vi "Create Minor Grid Lines.vi"(0 "Major Count":u16, 1 "Axis":enum16{"X-Axis", "Y-Axis", "Z-Axis"}(ring), 2 "Grid Plane Visible":T1, 5 "Minor Count":u16, 7 "Range":cluster{"Max":sgl, "Min":sgl}, 9 "Grid Color":u32(colorbox), 11 "error in (no error)":errorcluster, 12 "Inverted?":bool, 13 "Logarithm?":bool) -> (4 "Grid Object Out":refnum<vi>, 15 "error out":errorcluster)   [LabVIEW 2020, in "3D Plot.lvclass"]
uses:
  <vilib>/Math Plots/3D Math Plots/3D Plot/3D Plot/3D Plot.lvclass
  <vilib>/picture/3D Picture Control/Object/Create Object (name).vi
  <vilib>/picture/3D Picture Control/NI_3D Picture Control.lvlib
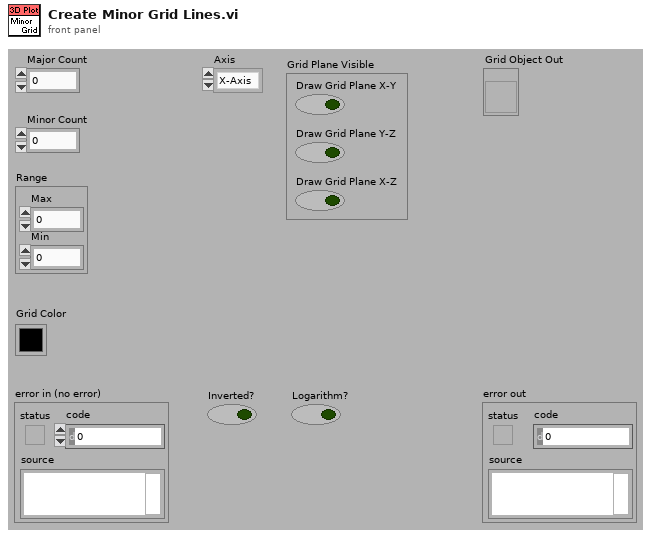
[diagram p1: front panel]
types:
  T1 = cluster{"Draw Grid Plane X-Y":bool, "Draw Grid Plane Y-Z":bool, "Draw Grid Plane X-Z":bool}
  T2 = enum16{"Overall", "Per Primitive", "Per Vertex", "Binding Off"}
  T3 = enum16{"Points", "Lines", "Line Strip", "Line Loop", "Triangles", "Triangle Strip", "Triangle Fan", "Quads", "Quad Strip", "Polygon"}
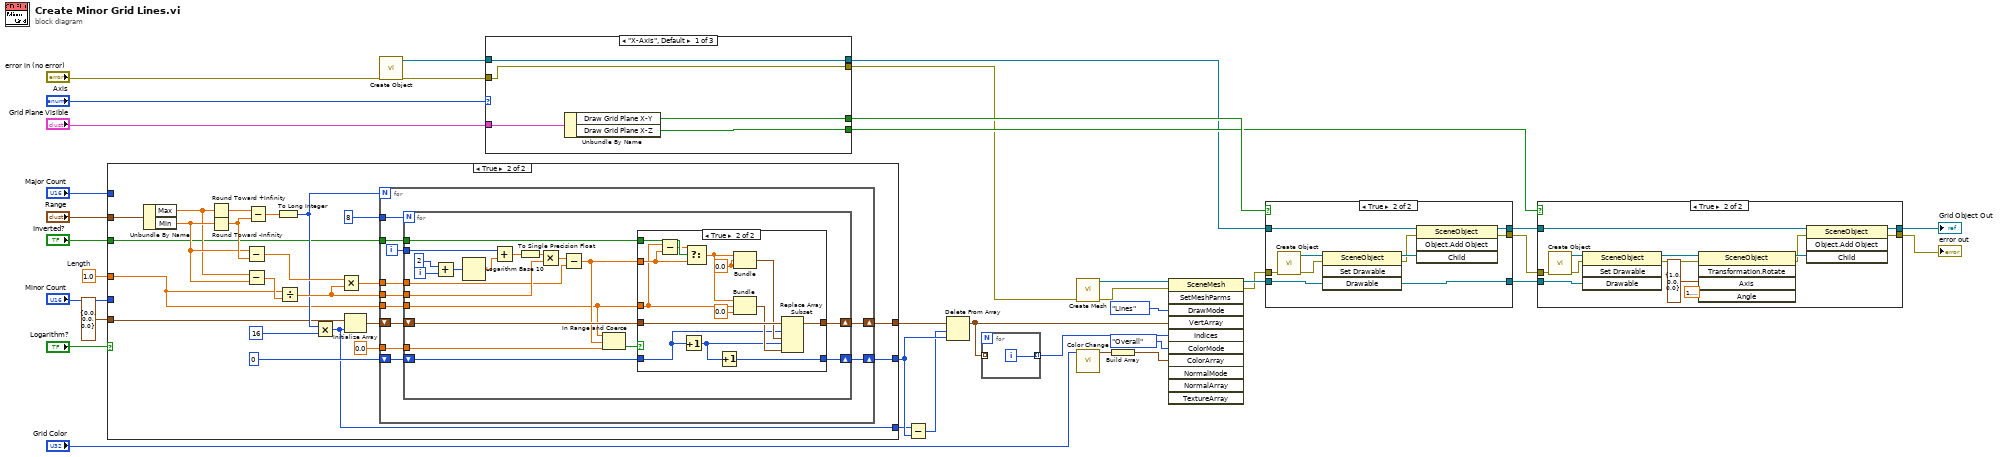
[diagram p0: block diagram]
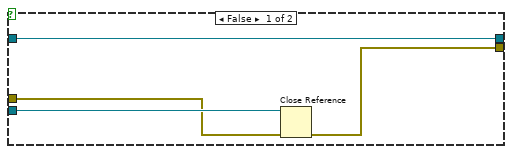
[diagram p2: hidden frame]
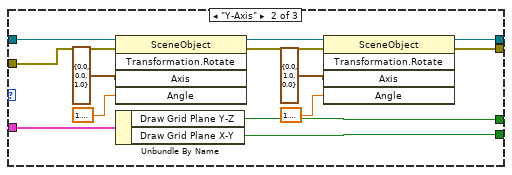
[diagram p3: hidden frame]
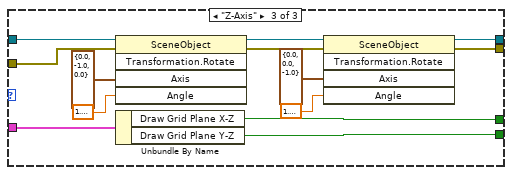
[diagram p4: hidden frame]
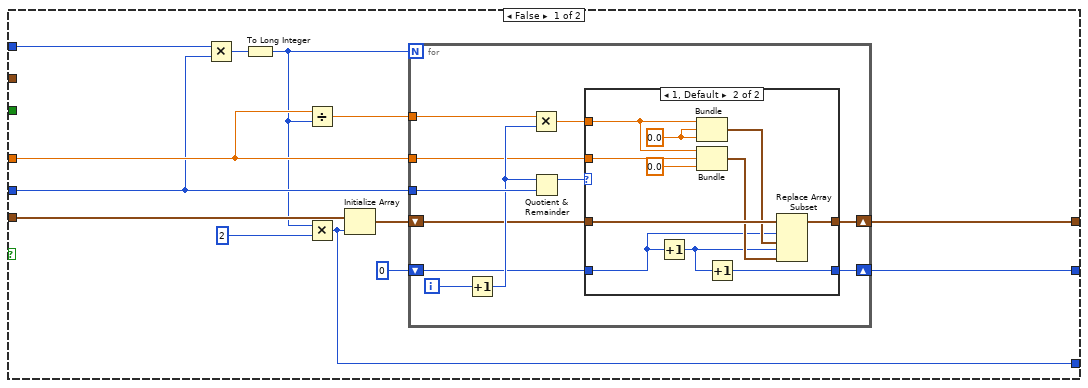
[diagram p6: hidden frame]
diagram:
  w36 = sgl 1.0  # Length
  n1 = case shown="True" "Logarithm?" {
    tunnel: w36 -> [w48 w78]
    tunnel: [w39 w76] -> w5
    tunnel: "Major Count" -> [w47 _]
    tunnel: "Minor Count" -> [w46 _]
    tunnel: "Range" -> [_ w80]
    tunnel: "Inverted?" -> [_ w79]
    tunnel: cluster{"X":sgl, "Y":sgl, "Z":sgl} {"X"=0.0, "Y"=0.0, "Z"=0.0} ("3D Point") -> [w45 w77]
    tunnel: [w38 w75] -> w3
    tunnel: [w37 w74] -> w1
    frame False {
      n2 = Multiply(x=w47, y=w46) -> (x*y=w41:u16)
      n3 = To Long Integer(number=w41) -> (32bit integer=w40:i32)
      n4 = Divide(x=w48, y=w40) -> (x/y=w49:sgl)
      n5 = Multiply(x=w40, y=2) -> (x*y=w37:i32)
      n6 = Initialize Array(w45, w37) -> (w44:cluster{"X":sgl, "Y":sgl, "Z":sgl}[])
      n7 = for {
        N: w40 -> [_]
        tunnel: w49 -> [w60]
        tunnel: w46 -> [w59]
        shift-right: [w53] -> w39
        shift-left: w44 -> [w54]
        tunnel: w48 -> [w52]
        shift-right: [w50] -> w38
        shift-left: 0 ("y") -> [w51]
        i -> [w57]
        n8 = Increment(x=w57) -> (x+1=w56:i32)
        n9 = Multiply(x=w60, y=w56) -> (x*y=w55:sgl)
        n10 = Quotient & Remainder(x=w56, y=w59) -> (x-y*floor(x/y)=w58:i32)  [unwired: 1 out]
        n11 = case shown="1, Default" w58 {
          tunnel: w55 -> [_ w71]
          tunnel: [w62 w68] -> w53
          tunnel: w54 -> [w62 w69]
          tunnel: w52 -> [_ w70]
          tunnel: w51 -> [w61 w65]
          tunnel: [w61 w63] -> w50
          frame 0 {
          }
          frame 1, Default {
            w72 = sgl 0.0
            n12 = Increment(x=w65) -> (x+1=w64:i32)
            n13 = Bundle(w71, w72, w72) -> (w67:cluster{sgl, sgl, sgl})  [unwired: 1 out]
            n14 = Bundle(w71, "Length"=w70, sgl 0.0) -> (w66:cluster{sgl, "Length":sgl, sgl})  [unwired: 1 out]
            n15 = Increment(x=w64) -> (x+1=w63:i32)
            n16 = Replace Array Subset(array=w69, new element #1=w67, index #1=w65, new element #2=w66, index #2=w64) -> (w68:cluster{"X":sgl, "Y":sgl, "Z":sgl}[])
          }
        }
      }
    }
    frame True {
      n17 = Unbundle By Name(w80) -> ("Max"=w87:sgl, "Min"=w90:sgl)
      n18 = Round Toward +Infinity(x=w87) -> (ceil(x): smallest int >= x=w86:sgl)
      n19 = Round Toward -Infinity(1:w90) -> (0:w91:sgl)
      n20 = Subtract(x=w90, y=w91) -> (x-y=w92:sgl)
      n21 = Subtract(x=w87, y=w90) -> (x-y=w88:sgl)
      n22 = Subtract(x=w86, y=w91) -> (x-y=w89:sgl)
      n23 = To Long Integer(number=w89) -> (32bit integer=w83:i32)
      n24 = Divide(x=w78, y=w88) -> (x/y=w95:sgl)
      n25 = Multiply(x=w83, y=16 ("x")) -> (x*y=w74:i32)
      n26 = Multiply(x=w92, y=w95) -> (x*y=w94:sgl)
      n27 = Initialize Array(w77, w74) -> (w81:cluster{"X":sgl, "Y":sgl, "Z":sgl}[])
      n28 = for {
        N: w83 -> [_]
        shift-right: [w105] -> w76
        shift-left: w81 -> [w106]
        tunnel: w78 -> [w104]
        tunnel: w95 -> [w103]
        tunnel: w79 -> [w101]
        tunnel: 8 -> [w100]
        shift-right: [w98] -> w75
        shift-left: 0 -> [w99]
        tunnel: w94 -> [w97]
        tunnel: sgl 0.0 ("lower limit") -> [w96]
        i -> [w102]
        n29 = for {
          N: w100 -> [_]
          tunnel: w102 -> [w122]
          shift-right: [w115] -> w105
          shift-left: w106 -> [w116]
          tunnel: w104 -> [w108]
          tunnel: w103 -> [w119]
          tunnel: w101 -> [w120]
          shift-right: [w114] -> w98
          shift-left: w99 -> [w113]
          tunnel: w97 -> [w111]
          tunnel: w96 -> [w107]
          i -> [w125]
          n30 = Add(x=2, y=w125) -> (x+y=w124:i32)
          n31 = Logarithm Base 10(1:w124) -> (0:w123:dbl)
          n32 = Add(x=w122, y=w123) -> (x+y=w118:dbl)
          n33 = To Single Precision Float(number=w118) -> (single precision float=w117:sgl)
          n34 = Multiply(x=w117, y=w119) -> (x*y=w112:sgl)
          n35 = Subtract(x=w112, y=w111) -> (x-y=w109:sgl)
          n36 = In Range and Coerce(upper limit=w108, x=w109, lower limit=w107) -> (In Range?=w110:bool)  [unwired: 1 out]
          n37 = case shown="True" w110 {
            tunnel: w120 -> [_ w141]
            tunnel: w109 -> [_ w139]
            tunnel: w108 -> [_ w135]
            tunnel: w116 -> [w127 w134]
            tunnel: [w127 w133] -> w115
            tunnel: [w126 w130] -> w114
            tunnel: w113 -> [w126 w128]
            frame False {
            }
            frame True {
              w138 = sgl 0.0
              n38 = Subtract(x=w135, y=w139) -> (x-y=w140:sgl)
              n39 = Increment(x=w128) -> (x+1=w129:i32)
              n40 = Select(t=w140, s=w141, f=w139) -> (s? t:f=w136:sgl)
              n41 = Increment(x=w129) -> (x+1=w130:i32)
              n42 = Bundle(w136, w138, w138) -> (w132:cluster{sgl, sgl, sgl})  [unwired: 1 out]
              n43 = Bundle(w136, "Length"=w135, sgl 0.0) -> (w131:cluster{sgl, "Length":sgl, sgl})  [unwired: 1 out]
              n44 = Replace Array Subset(array=w134, new element #1=w132, index #1=w128, new element #2=w131, index #2=w129) -> (w133:cluster{"X":sgl, "Y":sgl, "Z":sgl}[])
            }
          }
        }
      }
    }
  }
  n45 = call-poly <vilib>:"Create Object.vi"("error in (no error)"="error in (no error)") -> ("error out"=w15:errorcluster, "Scene:New Object"=w14:refnum<vi>)  [unwired: 9 in]
  n46 = case shown="\"X-Axis\", Default" "Axis" {
    tunnel: [w146 w150 w164] -> w13
    tunnel: w14 -> [w146 w153 w166]
    tunnel: [w145 w151 w165] -> w8
    tunnel: w15 -> [w145 w152 w163]
    tunnel: "Grid Plane Visible" -> [w144 w149 w162]
    tunnel: [w143 w148 w161] -> w16
    tunnel: [w142 w147 w160] -> w17
    frame "X-Axis", Default {
      n47 = Unbundle By Name(w144) -> ("Draw Grid Plane X-Y"=w142:bool, "Draw Grid Plane X-Z"=w143:bool)
    }
    frame "Y-Axis" {
      n48 = invoke class="SceneObject" method="Transformation.Rotate"(reference=w153, error in=w152, "Axis"=cluster{"X":sgl, "Y":sgl, "Z":sgl} {"X"=0.0, "Y"=0.0, "Z"=1.0}, "Angle"=1.5707963267948966) -> (reference out=w158:refnum<vi>, error out=w159:errorcluster)  [unwired: 1 in, 3 out]
      n49 = Unbundle By Name(w149) -> ("Draw Grid Plane Y-Z"=w147:bool, "Draw Grid Plane X-Y"=w148:bool)
      n50 = invoke class="SceneObject" method="Transformation.Rotate"(reference=w158, error in=w159, "Axis"=cluster{"X":sgl, "Y":sgl, "Z":sgl} {"X"=0.0, "Y"=1.0, "Z"=0.0}, "Angle"=1.5707963267948966) -> (reference out=w150:refnum<vi>, error out=w151:errorcluster)  [unwired: 1 in, 3 out]
    }
    frame "Z-Axis" {
      n51 = invoke class="SceneObject" method="Transformation.Rotate"(reference=w166, error in=w163, "Axis"=cluster{"X":sgl, "Y":sgl, "Z":sgl} {"X"=0.0, "Y"=-1.0, "Z"=0.0}, "Angle"=1.5707963267948966) -> (reference out=w167:refnum<vi>, error out=w172:errorcluster)  [unwired: 1 in, 3 out]
      n52 = Unbundle By Name(w162) -> ("Draw Grid Plane X-Z"=w160:bool, "Draw Grid Plane Y-Z"=w161:bool)
      n53 = invoke class="SceneObject" method="Transformation.Rotate"(reference=w167, error in=w172, "Axis"=cluster{"X":sgl, "Y":sgl, "Z":sgl} {"X"=0.0, "Y"=0.0, "Z"=-1.0}, "Angle"=1.5707963267948966) -> (reference out=w164:refnum<vi>, error out=w165:errorcluster)  [unwired: 1 in, 3 out]
    }
  }
  n54 = Subtract(x=w1, y=w3) -> (x-y=w2:i32)
  n55 = Delete From Array(array=w5, length=w2, index=w3) -> (array with subset deleted=w4:cluster{"X":sgl, "Y":sgl, "Z":sgl}[])  [unwired: 1 out]
  n56 = for {
    tunnel: [w173] -> w21 mode=indexing
    tunnel: w4 -> [_] mode=indexing
    i -> [w173]
  }
  n57 = call <vilib>:"Create Mesh.vi"("error in (no error)"=w8) -> ("error out"=w22:errorcluster, "New Mesh Refnum"=w24:refnum<vi>)  [unwired: 9 out]
  n58 = call <vilib>:"Color Change.vi"("Color"="Grid Color") -> ("RGBA"=w18:cluster{"R":sgl, "G":sgl, "B":sgl, "A":sgl})  [unwired: 1 in, 9 out]
  n59 = Build Array(w18) -> (w20:cluster{"R":sgl, "G":sgl, "B":sgl, "A":sgl}[])
  n60 = invoke class="SceneMesh" method="SetMeshParms"(reference=w24, error in=w22, "DrawMode"=T3."Lines" ("Draw Mode"), "VertArray"=w4, "Indices"=w21, "ColorMode"=T2."Overall" ("Color Binding Mode"), "ColorArray"=w20) -> (reference out=w9:refnum<vi>, error out=w7:errorcluster)  [unwired: 4 in, 9 out]
  n61 = case shown="True" w17 {
    tunnel: w9 -> [w174 w185]
    tunnel: [w174 w183] -> w12
    tunnel: [w175 w177] -> w10
    tunnel: [w176 w181] -> w11
    tunnel: w13 -> [w176 w180]
    tunnel: w7 -> [w175 w179]
    frame False {
    }
    frame True {
      n62 = call-poly <vilib>:"Create Object.vi"("error in (no error)"=w179) -> ("error out"=w186:errorcluster, "Scene:New Object"=w184:refnum<vi>)  [unwired: 9 in]
      n63 = invoke class="SceneObject" method="Set Drawable"(reference=w184, error in=w186, "Drawable"=w185) -> (reference out=w182:refnum<vi>, error out=w178:errorcluster, "Drawable"=w183:refnum<vi>)  [unwired: 1 in, 1 out]
      n64 = invoke class="SceneObject" method="Object.Add Object"(reference=w180, error in=w178, "Child"=w182) -> (reference out=w181:refnum<vi>, error out=w177:errorcluster)  [unwired: 1 in, 2 out]
    }
  }
  n65 = case shown="True" w16 {
    tunnel: w10 -> [w188 w201]
    tunnel: w11 -> [w190 w200]
    tunnel: [w190 w199] -> w27
    tunnel: [w187 w198] -> w28
    tunnel: w12 -> [w189 w194]
    frame False {
      n66 = Close Reference(reference=w189, error in (no error)=w188) -> (error out=w187:errorcluster)
    }
    frame True {
      n67 = call-poly <vilib>:"Create Object.vi"("error in (no error)"=w201) -> ("error out"=w195:errorcluster, "Scene:New Object"=w196:refnum<vi>)  [unwired: 9 in]
      n68 = invoke class="SceneObject" method="Set Drawable"(reference=w196, error in=w195, "Drawable"=w194) -> (reference out=w193:refnum<vi>, error out=w192:errorcluster)  [unwired: 1 in, 2 out]
      n69 = invoke class="SceneObject" method="Transformation.Rotate"(reference=w193, error in=w192, "Axis"=cluster{"X":sgl, "Y":sgl, "Z":sgl} {"X"=1.0, "Y"=0.0, "Z"=0.0}, "Angle"=sgl 1.5707964) -> (reference out=w197:refnum<vi>, error out=w191:errorcluster)  [unwired: 1 in, 3 out]
      n70 = invoke class="SceneObject" method="Object.Add Object"(reference=w200, error in=w191, "Child"=w197) -> (reference out=w199:refnum<vi>, error out=w198:errorcluster)  [unwired: 1 in, 2 out]
    }
  }
  "Grid Object Out" <- w27
  "error out" <- w28
